vi "Instrument.OxfordVRM.Client.vi"(8 "error in (no error)":errorcluster, 9 "Data":variant, 10 "Commands":T1, 11 "Instrument.VRM in":refnum<class "Instrument.OxfordVRM.lvclass">) -> (0 "error out":errorcluster, 1 "Data out":variant, 3 "Instrument.VRM out":refnum<class "Instrument.OxfordVRM.lvclass">)   [LabVIEW 2016, in "Instrument.OxfordVRM.lvclass"]
uses:
  Instrument.OxfordVRM.lvclass
  C:/Program Files (x86)/National Instruments/LabVIEW 2016/user.lib/LevyLab/Levylab Instruments/SMOs/Instrument/Instrument.lvclass
  Typedefs/Instrument.VRM.Commands-enum.ctl
  <userlib>/LevyLab/Levylab Instruments/SMOs/Instrument/Instrument.lvclass
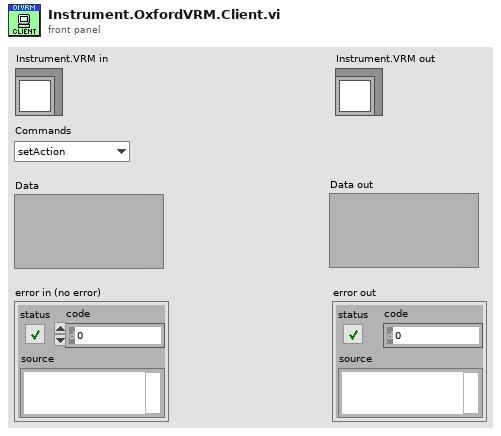
[diagram p1: front panel]
types:
  T1 = typedef "Instrument.OxfordVRM.lvclass/Instrument.VRM.Commands-enum.ctl" = enum16{"setAction", "setTarget", "setMagnetField", "getStatus", "getTarget", "getMagnetField"}
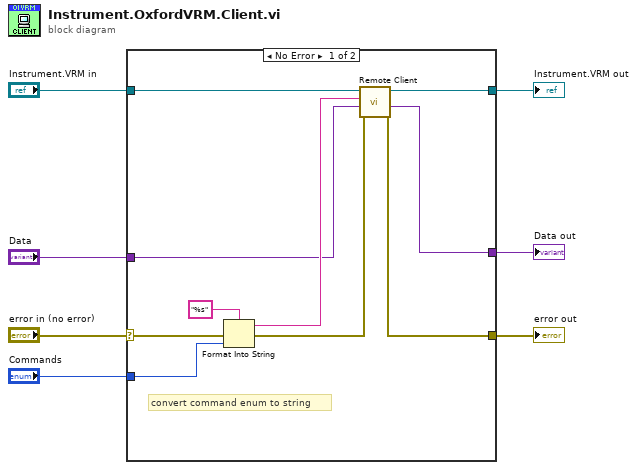
[diagram p0: block diagram]
diagram:
  n1 = case shown="No Error" "error in (no error)" {
    selector: "error in (no error)" -> [w11 w19]
    tunnel: "Data" -> [w9 _]
    tunnel: [w14 w19] -> w6
    tunnel: [w13 _] -> w5
    tunnel: "Commands" -> [w8 _]
    tunnel: "Instrument.VRM in" -> [w16 w18]
    tunnel: [w15 w18] -> w1
    frame No Error {
      # "convert command enum to string"
      n2 = Format Into String(format string="%s", error in=w11, w8) -> (resulting string=w10:string, error out=w12:errorcluster)  [unwired: 1 in]
      n3 = call <userlib>:"Remote Client.vi"("error in (no error)"=w12, "Data"=w9, "Command"=w10, "Instrument in"=w16) -> ("error out"=w14:errorcluster, "Data out"=w13:variant, "Instrument out"=w15:refnum<class "Instrument.OxfordVRM.lvclass">)  [unwired: 4 in, 1 out]
    }
    frame Error {
    }
  }
  "Instrument.VRM out" <- w1
  "error out" <- w6
  "Data out" <- w5
